vi "ClearFaults.vi"(11 "Engine_1DO_2DI in":refnum<class "Engine_1DO_2DI.lvclass">) -> (3 "Engine_1DO_2DI out":refnum<class "Engine_1DO_2DI.lvclass">)   [LabVIEW 2019, in "Engine_1DO_2DI.lvclass"]
uses:
  Engine_1DO_2DI.lvclass
  Engine_1DO_2DI.lvclass/Engine_1DO_2DI.ctl
  DA_class/DA.lvclass
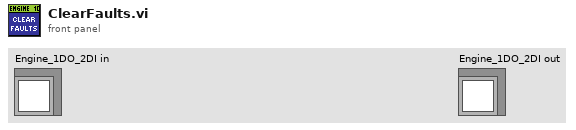
[diagram p1: front panel]
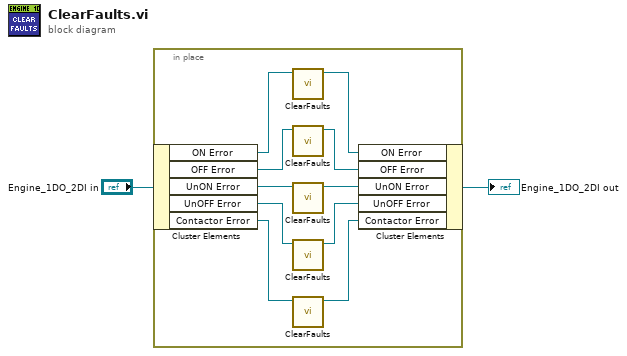
[diagram p0: block diagram]
diagram:
  n1 = in-place {
    n2 = in-place-cluster #1("Engine_1DO_2DI in") -> ("ON Error"=w12:refnum<class "DA.lvclass">, "OFF Error"=w10:refnum<class "DA.lvclass">, "UnON Error"=w9:refnum<class "DA.lvclass">, "UnOFF Error"=w8:refnum<class "DA.lvclass">, "Contactor Error"=w7:refnum<class "DA.lvclass">)
    n3 = call-dynamic "ClearFaults.vi"("DA in"=w12) -> ("DA out"=w11:refnum<class "DA.lvclass">)  [unwired: 10 in]
    n4 = call-dynamic "ClearFaults.vi"("DA in"=w10) -> ("DA out"=w6:refnum<class "DA.lvclass">)  [unwired: 10 in]
    n5 = call-dynamic "ClearFaults.vi"("DA in"=w9) -> ("DA out"=w5:refnum<class "DA.lvclass">)  [unwired: 10 in]
    n6 = call-dynamic "ClearFaults.vi"("DA in"=w8) -> ("DA out"=w4:refnum<class "DA.lvclass">)  [unwired: 10 in]
    n7 = call-dynamic "ClearFaults.vi"("DA in"=w7) -> ("DA out"=w3:refnum<class "DA.lvclass">)  [unwired: 10 in]
    n8 = in-place-cluster #1("ON Error"=w11, "OFF Error"=w6, "UnON Error"=w5, "UnOFF Error"=w4, "Contactor Error"=w3) -> (→"Engine_1DO_2DI out":refnum<class "Engine_1DO_2DI.lvclass">)
  }
